vi "Deform Array Increment Limiter Demo.vi"(8 "Increment Array":dbl[](array[numeric])=[0.1, 0.05, 0.1], 11 "Defrom Ref":dbl[](array[numeric])=[1.0, 1.0, 1.0, 0.0, 0.0, 0.0, 0.0, 0.0, 0.0]) -> (3 "Deform Output":dbl[](array[numeric]))   [LabVIEW 2016]
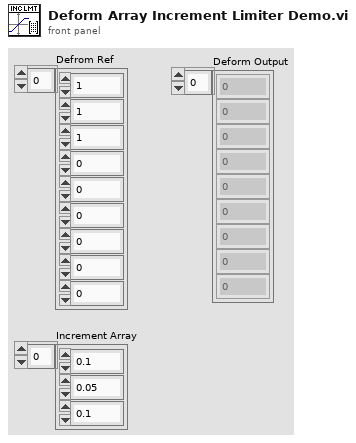
[diagram p1: front panel]
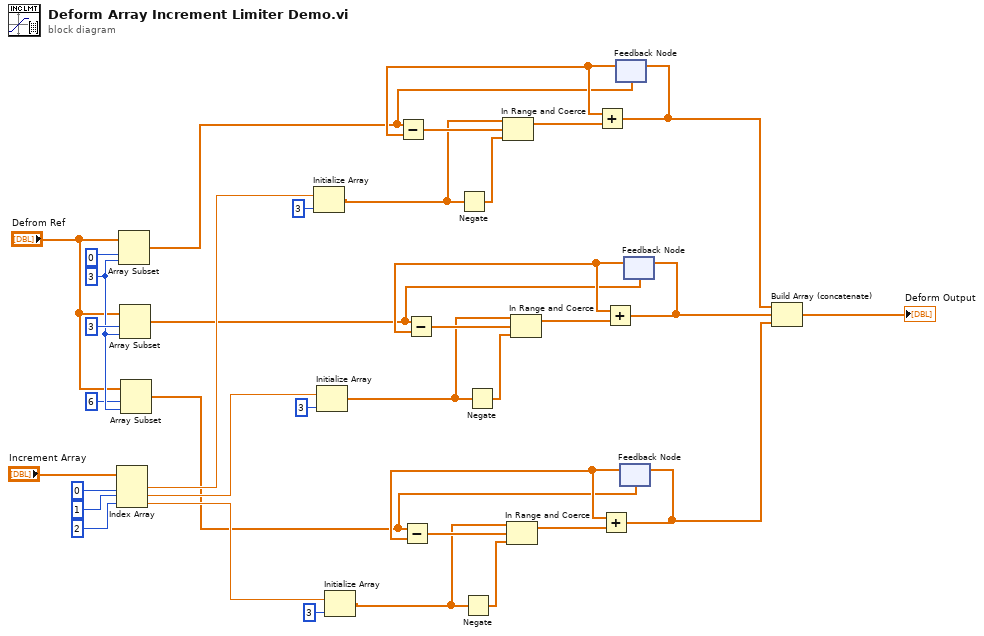
[diagram p0: block diagram]
diagram:
  w31 = 3 ("length")
  n1 = Index Array(array="Increment Array", index #1=0 ("index"), index #2=1 ("index"), index #3=2 ("index")) -> (element #1=w13:dbl, element #2=w11:dbl, element #3=w9:dbl)
  n2 = Array Subset(array="Defrom Ref", index=0, length=w31) -> (w7:dbl[])
  n3 = Array Subset(array="Defrom Ref", index=3, length=w31) -> (w6:dbl[])
  n4 = Array Subset(array="Defrom Ref", index=6, length=w31) -> (w5:dbl[])
  n5 = Initialize Array(w13, 3 ("dimension size")) -> (w12:dbl[])
  n6 = Initialize Array(w11, 3 ("dimension size")) -> (w10:dbl[])
  n7 = Initialize Array(w9, 3 ("dimension size")) -> (w8:dbl[])
  n8 = Negate(x=w12) -> (-x=w37:dbl[])
  n9 = Negate(x=w8) -> (-x=w20:dbl[])
  n10 = Negate(x=w10) -> (-x=w21:dbl[])
  n11 = feedback #1(w7) -> (w35:dbl[])
  n12 = Subtract(x=w7, y=w35) -> (x-y=w34:dbl[])
  n13 = In Range and Coerce(upper limit=w12, x=w34, lower limit=w37) -> (coerced(x)=w36:dbl[])  [unwired: 1 out]
  n14 = Add(x=w35, y=w36) -> (x+y=w4:dbl[])
  n15 = feedback-in #1(w4) -> ()
  n16 = feedback #2(w5) -> (w18:dbl[])
  n17 = Subtract(x=w5, y=w18) -> (x-y=w17:dbl[])
  n18 = In Range and Coerce(upper limit=w8, x=w17, lower limit=w20) -> (coerced(x)=w19:dbl[])  [unwired: 1 out]
  n19 = Add(x=w18, y=w19) -> (x+y=w2:dbl[])
  n20 = feedback-in #2(w2) -> ()
  n21 = feedback #3(w6) -> (w23:dbl[])
  n22 = Subtract(x=w6, y=w23) -> (x-y=w24:dbl[])
  n23 = In Range and Coerce(upper limit=w10, x=w24, lower limit=w21) -> (coerced(x)=w22:dbl[])  [unwired: 1 out]
  n24 = Add(x=w23, y=w22) -> (x+y=w3:dbl[])
  n25 = feedback-in #3(w3) -> ()
  n26 = Build Array (concatenate)(w4, w3, w2) -> (→"Deform Output":dbl[])
